vi "ex3.vi"() -> ()   [LabVIEW 2022 SP3]
panel:
  out "replaced substring":string
  in  "given number":i32
  in  "Name":string
  in  "Enum":enum16{"ClearList", "GetList", "AddRecord"}(ring)
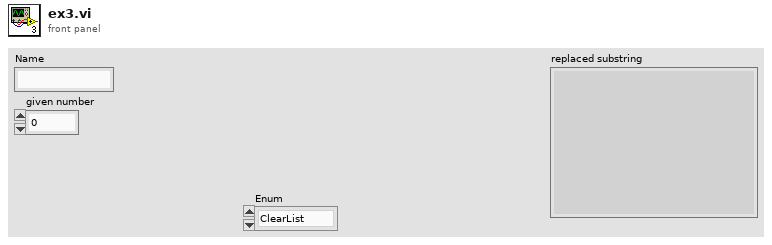
[diagram p1: front panel]
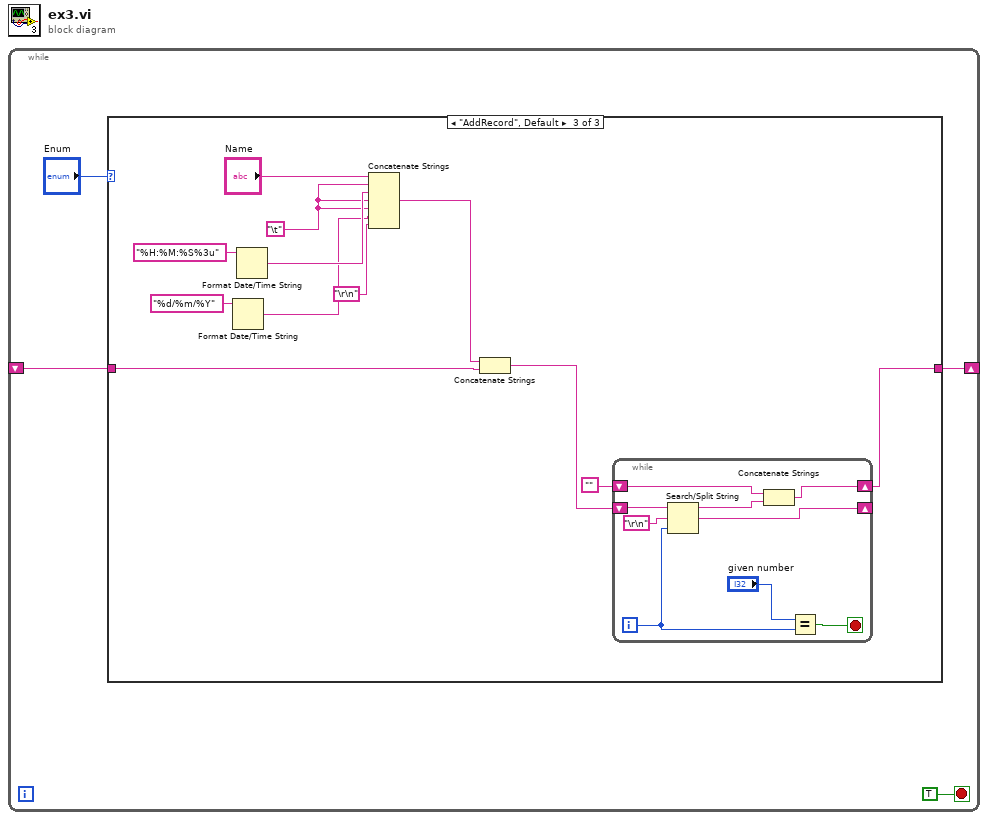
[diagram p0: block diagram]
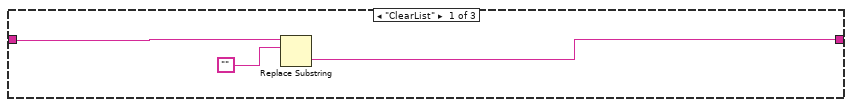
[diagram p2: hidden frame]
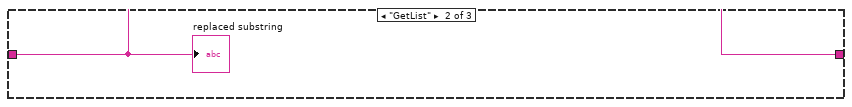
[diagram p3: hidden frame]
diagram:
  n1 = while {
    shift-right: [w1] -> _
    shift-left: _ -> [w3]
    stop <- TRUE stop-if-true
    n2 = case shown="\"AddRecord\", Default" "Enum" {
      tunnel: w3 -> [w7 w8 w12]
      tunnel: [w5 w8 w9] -> w1
      frame "ClearList" {
        n3 = Replace Substring(4:"", 5:w7) -> (0:w5:string)  [unwired: 2 in, 1 out]
      }
      frame "GetList" {
        "replaced substring" <- w8
      }
      frame "AddRecord", Default {
        w16 = "\t"
        n4 = Format Date/Time String(time format string (%c)="%d/%m/%Y") -> (date/time string=w15:string)  [unwired: 2 in]
        n5 = Format Date/Time String(time format string (%c)="%H:%M:%S%3u") -> (date/time string=w17:string)  [unwired: 2 in]
        n6 = Concatenate Strings("Name", w16, w17, w16, w16, w15, "\r\n") -> (w13:string)
        n7 = Concatenate Strings(w13, w12) -> (w11:string)
        n8 = while {
          shift-right: [w21] -> _
          shift-left: w11 -> [w29]
          shift-right: [w22] -> w9
          shift-left: "" -> [w23]
          i -> [w27]
          stop <- w25 stop-if-true
          n9 = Search/Split String(string=w29, search string/char (-)="\r\n", offset (0)=w27) -> (substring before match=w24:string, match + rest of string=w21:string)  [unwired: 1 out]
          n10 = Concatenate Strings(w23, w24) -> (w22:string)
          n11 = Equal?(x="given number", y=w27) -> (x = y?=w25:bool)
        }
      }
    }
  }
